vi "Read SnP File (S1P).vi"(0 "S1P File Path":path, 11 "Error In":errorcluster) -> (4 "S-parameters":cdb[](array[numeric]) format="%#.6g", 6 "Frequencies (Hz)":dbl[](array[numeric]), 8 "Z0 (Ohm)":cdb, 15 "Error Out":errorcluster)   [LabVIEW 2023, in "NI_HFNetworkAnalysis.lvlib"]
doc: "Reads 1-port S-parameters from the specified file assuming Touchstone File Format specifications.\n\n<b>Known limitation :</b>\nSupport for S-parameter data only."
uses:
  NI_HFNetworkAnalysis.lvlib
  C:/srd-semi-rfcal-software/AuxTools/STSRFFixtureCharactUtility/Source/Code Modules/Fixture/Dependencies/HFNetworkAnalysis/Support Files/NACE.Utils.Data.dll
  Support Files/NACE.Utils.Data.dll
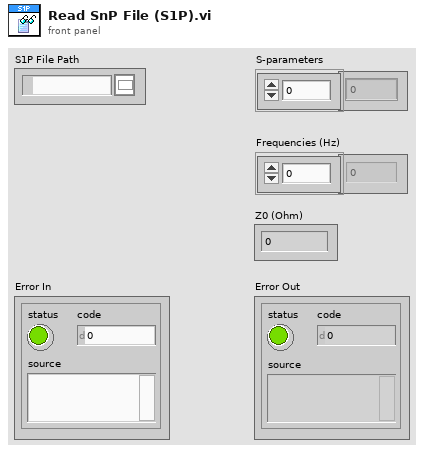
[diagram p1: front panel]
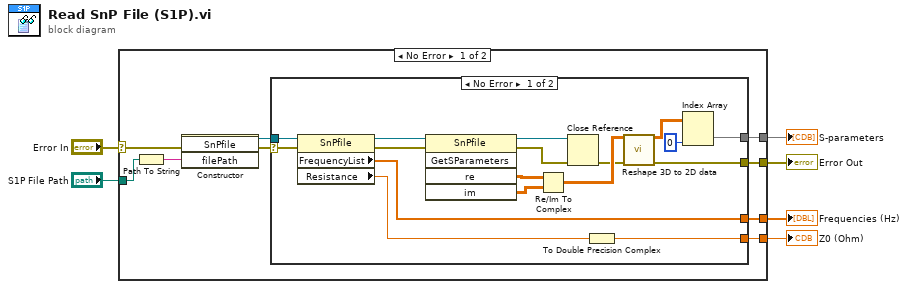
[diagram p0: block diagram]
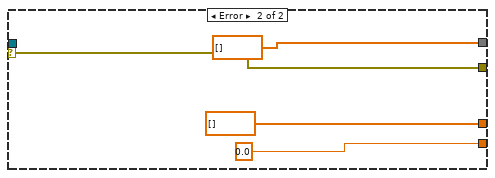
[diagram p2: hidden frame]
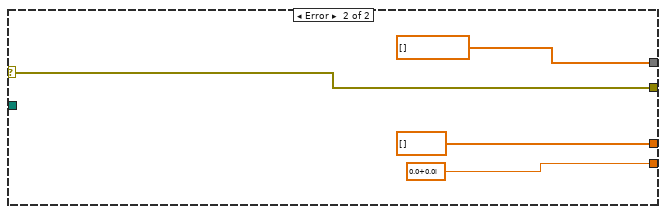
[diagram p3: hidden frame]
diagram:
  n1 = case shown="No Error" "Error In" {
    selector: "Error In" -> [w11 w40]
    tunnel: [w10 w40] -> w5
    tunnel: "S1P File Path" -> [w12 _]
    tunnel: [w9 dbl[] [] ("FrequencyList")] -> w3
    tunnel: [w8 cdb 0.0+0.0i ("Resistance")] -> w2
    tunnel: [w7 cdb[] [] ("Parameters Out (2D)")] -> w1
    frame No Error {
      n2 = Path To String(path=w12) -> (string=w13:string)
      n3 = constructor class="SnPfile"(error in=w11, "filePath"=w13) -> (reference out=w14:refnum<k24>, error out=w15:errorcluster)  [unwired: 2 in, 2 out]
      n4 = case shown="No Error" w15 {
        selector: w15 -> [w31 w34]
        tunnel: w14 -> [w32 _]
        tunnel: [w25 dbl[] [] ("FrequencyList")] -> w9
        tunnel: [w24 0.0 ("Resistance")] -> w8
        tunnel: [w19 w34] -> w10
        tunnel: [w18 cdb[] [] ("FrequencyList")] -> w7
        frame No Error {
          n5 = property class="SnPfile"(reference=w32, error in=w31) -> (reference out=w30:refnum<k24>, error out=w29:errorcluster, "FrequencyList"=w25:dbl[], "Resistance"=w26:dbl)
          n6 = invoke class="SnPfile" method="GetSParameters"(reference=w30, error in=w29) -> (reference out=w16:refnum<k24>, error out=w23:errorcluster, "re"=w28:dbl[][][], "im"=w27:dbl[][][])  [unwired: 3 in, 1 out]
          n7 = Re/Im To Complex(1:w27, 2:w28) -> (0:w22:cdb[][][])
          n8 = Close Reference(reference=w16, error in (no error)=w23) -> (error out=w17:errorcluster)
          n9 = To Double Precision Complex(1:w26) -> (0:w24:cdb)
          n10 = call "Reshape 3D to 2D data.vi"("Parameters In (3D)"=w22, "Error In"=w17) -> ("Parameters Out (2D)"=w21:cdb[][], "Error Out"=w19:errorcluster)  [unwired: 12 in]
          n11 = Index Array(array=w21, index (col)=0 ("disabled index (col)")) -> (element=w18:cdb[])  [unwired: 1 in]
        }
        frame Error {
        }
      }
    }
    frame Error {
    }
  }
  "Error Out" <- w5
  "S-parameters" <- w1
  "Frequencies (Hz)" <- w3
  "Z0 (Ohm)" <- w2
